vi "PSK_Mod_Demod_test.vi"() -> ()   [LabVIEW 2014]
uses:
  <vilib>/addons/Modulation/Digital/General/MT Generate Bits (Galois, PN Order).vi
  <vilib>/addons/Modulation/Digital/Support/Common/Validators/mod_Generate Bits Validate.vi
  <vilib>/addons/Modulation/Analog/support/mod_Set Error Source.vi
  <vilib>/addons/Modulation/Digital/General/MT Generate PSK System Parameters(M).vi
  <vilib>/addons/Modulation/Digital/Support/Common/Validators/mod_Generate Filter Coefficients Validate.vi
  <vilib>/addons/Modulation/Digital/General/subVIs/mod_Generate Filter Coefficients.vi
  <vilib>/addons/Modulation/Digital/General/subVIs/mod_Generate Bits PN Sequence.vi
  <vilib>/addons/Modulation/Digital/General/MT Generate PSK Synchronization Parameters (bit array).vi
  <vilib>/addons/Modulation/Digital/General/MT Map Bits to PSK Symbols.vi
  <vilib>/addons/Modulation/Digital/General/MT Generate Bits (User Defined).vi
  <vilib>/addons/Modulation/niDMT.lvlib
  <vilib>/addons/Modulation/niAMT.lvlib
panel:
  out "Before demod&compensation":waveform(dbl)(graph)
  out "After compensation&demod":waveform(dbl)(graph)
  out "logical AND":bool
  out "output bit stream 2":i8[](array[numeric]) caption="output bit stream"
  out "symbols":cdb[](array[numeric]) format="%.3f"
  in  "synchronization parameters":T1={"expected sync location (symbols)"=-1, "sync sequence"=[], "sync location uncertainty (symbols)"=0, "sync indent (symbols)"=0} {"sync sequence" format="%.2f"}
  out "bits received 2":i32
  out "output bit stream 3":i8[](array[numeric]) caption="output bit stream"
  in  "user base bit pattern":i8[](array[numeric]) caption="Input bit stream"
  out "bits received":i32
  out "bits sent":i32
  out "sync found index (symbols)":dbl format="%.4f"
  in  "IQ Sampling\nRate [S/sec]":dbl=500000.0 format="%#.6p"
  out "Constellation Graph":T2(graph) caption="Tx Signal Constellation"
  out "input bit stream":i8[](array[numeric]) caption="output bit stream"
  in  "filter parameters":T3={"Alpha"=0.5, "Filter Length"=6, "TX Filter"=enum."Root Raised Cos"} {"Alpha" format="%.2f"}
  in  "QPSK System Parameters":T4={"Samples per Symbol"=8, "symbol map"=[], "Differential PSK"=enum."disable", "PSK type"=0} {"PSK type" items=["normal", "shifted", "offset"]; "symbol map" format="%.3f"}
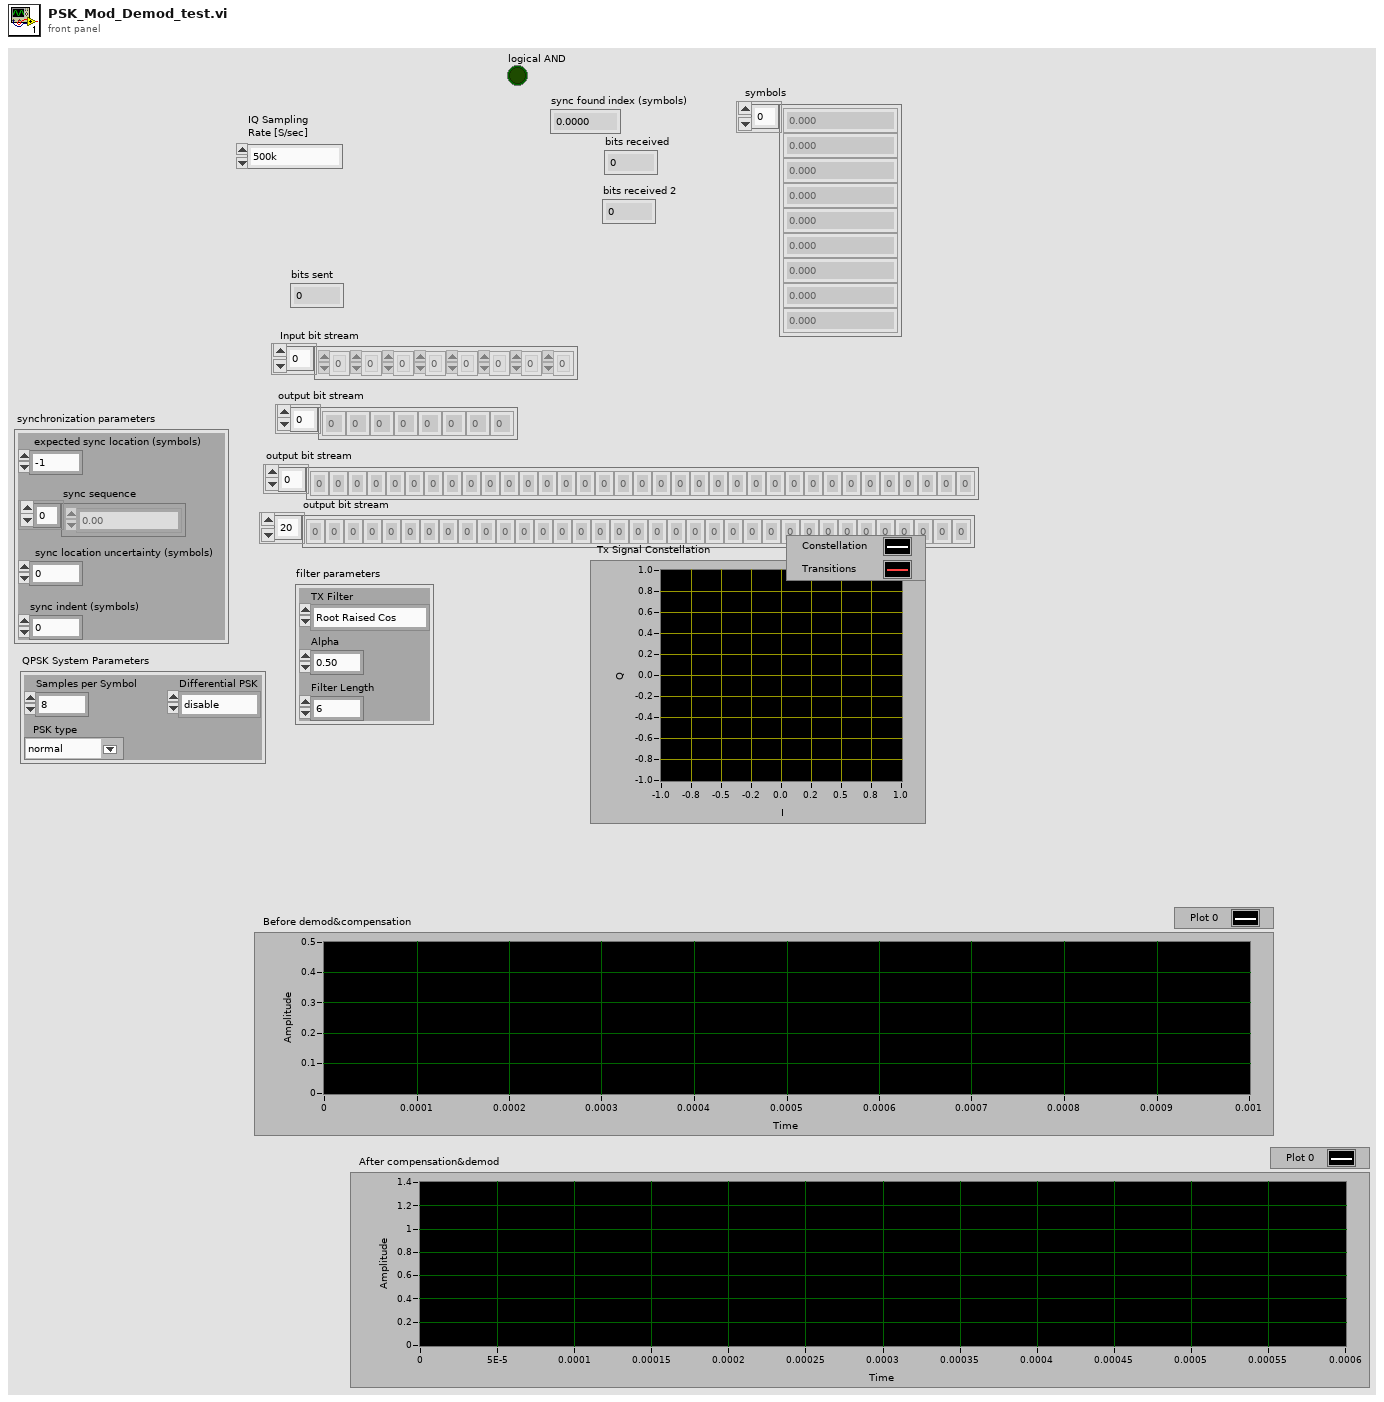
[diagram p1: front panel]
types:
  T1 = cluster{"expected sync location (symbols)":i32, "sync sequence":cdb[], "sync location uncertainty (symbols)":i32, "sync indent (symbols)":i32}
  T2 = cluster{"constellation":dbl[], "oversampled data":dbl[]}[]
  T3 = cluster{"Alpha":dbl, "Filter Length":i32, "TX Filter":enum16{"none", "Raised Cosine", "Root Raised Cos", "Gaussian"}}
  T4 = cluster{"Samples per Symbol":i32, "symbol map":cdb[], "Differential PSK":enum16{"disable", "enable"}, "PSK type":u16}
  T5 = enum16{"FSK", "PSK", "QAM", "MSK", "PAM", "ASK", "CPM"}
  T6 = enum16{"none", "Raised Cosine", "Root Raised Cos", "Gaussian"}
  T7 = cluster{"samples per symbol (16)":i32, "symbol map":cdb[], "differential PSK":enum16{"disable", "enable"}, "PSK type":u16}
  T8 = typedef "niAMT.lvlib/Complex Data Waveform.ctl" = cluster{"t0":dbl, "dt":dbl, "Y":cdb[]}
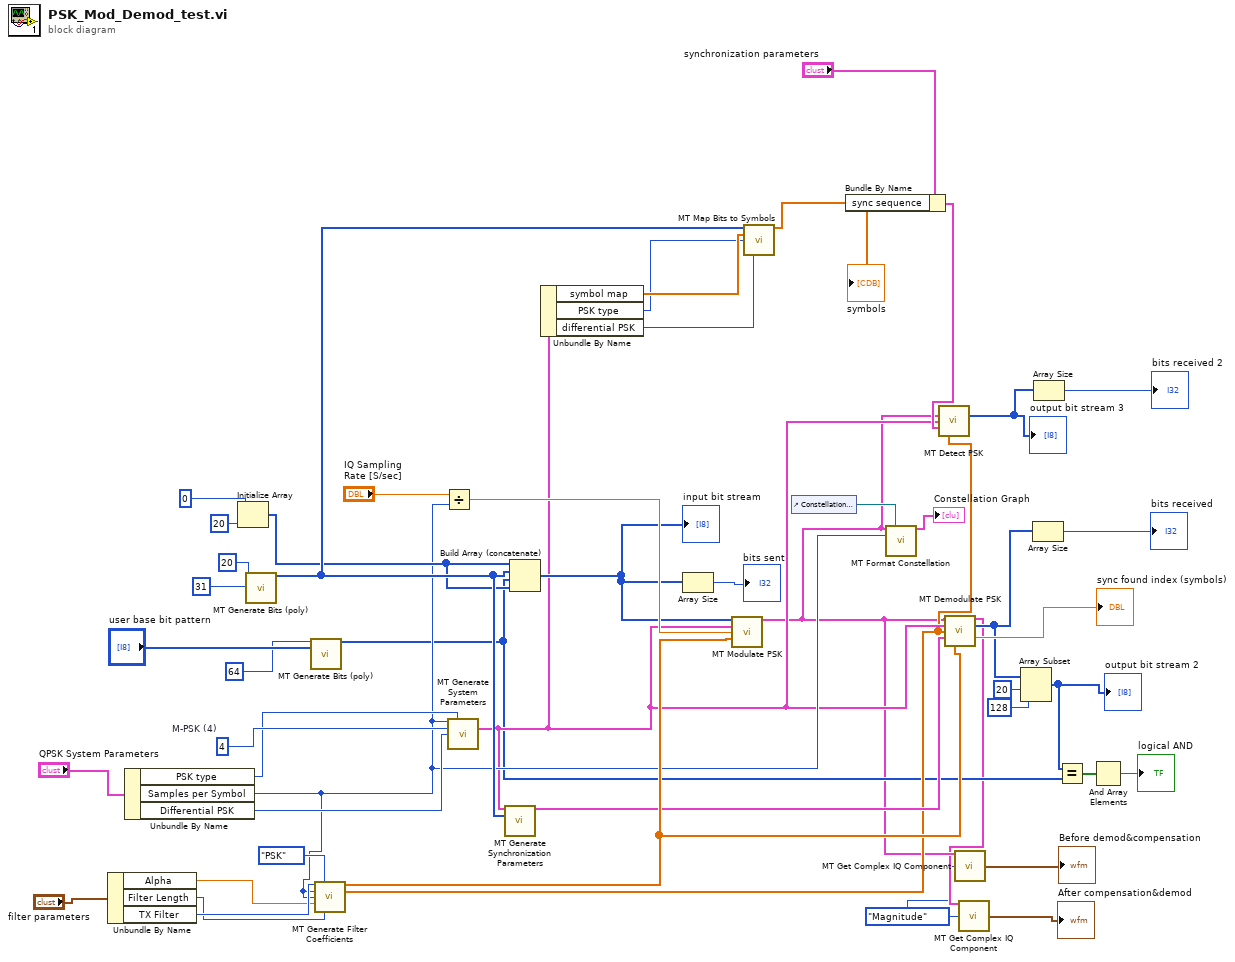
[diagram p0: block diagram]
diagram:
  w4 = enum16{"I", "Q", "Magnitude", "Phase"}."Magnitude" ("component choice")
  w48 = 4  # M-PSK (4)
  n1 = Unbundle By Name("filter parameters") -> ("Alpha"=w44:dbl, "Filter Length"=w45:i32, "TX Filter"=w46:T6)
  n2 = Unbundle By Name("QPSK System Parameters") -> ("PSK type"=w47:u16, "Samples per Symbol"=w16:i32, "Differential PSK"=w49:enum16{"disable", "enable"})
  n3 = Initialize Array(i8 0 ("element"), 20 ("dimension size")) -> (w18:i8[])
  n4 = call-poly <vilib>:"MT Generate Bits (poly).vi"("total bits (128)"=20, "PN sequence order (9)"=31) -> ("output bit stream"=w19:i8[])  [unwired: 11 in, 2 out]
  n5 = call-poly <vilib>:"MT Generate Bits (poly).vi"("total bits (128)"=64, "user base bit pattern"="user base bit pattern") -> ("output bit stream"=w9:i8[])  [unwired: 12 in, 1 out]
  n6 = call <vilib>:"MT Generate Filter Coefficients.vi"("pulse shaping filter (none)"=w46, "modulation type"=T5."PSK", "pulse shaping samples per symbol (16)"=w16, "matched samples per symbol (16)"=w16, "filter parameter"=w44, "filter length (symbols)"=w45) -> ("pulse shaping filter coefficients"=w41:dbl[], "matched filter coefficients"=w14:dbl[])  [unwired: 7 in, 1 out]
  n7 = Divide(x="IQ Sampling\nRate [S/sec]", y=w16) -> (x/y=w40:dbl)
  n8 = call-poly <vilib>:"MT Generate System Parameters.vi"("samples per symbol (16)"=w16, "PSK type"=w47, "M-PSK (4)"=w48, "differential PSK"=w49) -> ("PSK system parameters"=w15:T7)  [unwired: 9 in, 2 out]
  n9 = call-poly <vilib>:"MT Generate Synchronization Parameters.vi"("PSK system parameters"=w15, "sync bits"=w19) -> ("PSK synchronization parameters"=w17:T1)  [unwired: 12 in, 1 out]
  n10 = Build Array (concatenate)(w18, w19, w9, w18) -> (w33:i8[])
  "input bit stream" <- w33
  n11 = Unbundle By Name(w15) -> ("symbol map"=w23:cdb[], "PSK type"=w22:u16, "differential PSK"=w21:enum16{"disable", "enable"})
  n12 = Array Size(array=w33) -> (size(s)=→"bits sent":i32)
  n13 = call <vilib>:"MT Modulate PSK.vi"("input bit stream"=w33, "PSK system parameters"=w15, "symbol rate (Hz)"=w40, "pulse shaping filter coefficients"=w41) -> ("output complex waveform"=w6:T8)  [unwired: 9 in, 2 out]
  n14 = call-poly <vilib>:"MT Map Bits to Symbols.vi"("input bit stream"=w19, "symbol map"=w23, "PSK type"=w22, "differential PSK"=w21) -> ("symbols"=w24:cdb[])  [unwired: 10 in, 1 out]
  "symbols" <- w24
  n15 = control-ref of="Constellation Graph"() -> (w39:refnum<vi>)
  n16 = Bundle By Name(cluster="synchronization parameters", "sync sequence"=w24) -> (w25:T1)
  n17 = call <vilib>:"MT Format Constellation.vi"("waveform"=w6, "constellation reference"=w39, "samples per symbol"=w16) -> ("constellation graph"=→"Constellation Graph":T2)  [unwired: 11 in, 1 out]
  n18 = call <vilib>:"MT Detect PSK.vi"("input complex waveform"=w6, "PSK system parameters"=w15, "synchronization parameters"=w25, "matched filter coefficients"=w14) -> ("output bit stream"=w28:i8[])  [unwired: 9 in, 2 out]
  "output bit stream 3" <- w28
  n19 = call <vilib>:"MT Demodulate PSK.vi"("input complex waveform"=w6, "PSK system parameters"=w15, "matched filter coefficients"=w14, "synchronization parameters"=w17, "pulse shaping filter coefficients"=w41) -> ("recovered complex waveform"=w5:T8, "output bit stream"=w13:i8[], "sync found index (symbols)"=→"sync found index (symbols)":dbl)  [unwired: 6 in, 2 out]
  n20 = call <vilib>:"MT Get Complex IQ Component.vi"("IQ data (complex) in"=w6, "component choice"=w4) -> ("CE component"=→"Before demod&compensation":waveform(dbl))  [unwired: 11 in, 2 out]
  n21 = call <vilib>:"MT Get Complex IQ Component.vi"("IQ data (complex) in"=w5, "component choice"=w4) -> ("CE component"=→"After compensation&demod":waveform(dbl))  [unwired: 11 in, 2 out]
  n22 = Array Subset(array=w13, index=20, length=128) -> (w10:i8[])
  "output bit stream 2" <- w10
  n23 = Array Size(array=w13) -> (size(s)=→"bits received":i32)
  n24 = Array Size(array=w28) -> (size(s)=→"bits received 2":i32)
  n25 = Equal?(x=w10, y=w9) -> (x = y?=w8:bool[])
  n26 = And Array Elements(Boolean array=w8) -> (logical AND=→"logical AND":bool)
